vi "VSS_SimulatorCommand.vi"(11 "our_robots":T1[](array[typedef])) -> (2 "Array":u8[](array[numeric]))   [LabVIEW 2017]
uses:
  Core/AI Robot.ctl
  Intel/Functions Enum.ctl
  Intel/AttackerStates.ctl
  Path Planning/RRT/PathDests.ctl
  Path Planning/RRT/PathDest.ctl
panel:
  in  "k":dbl=10.0 format="%#_13g"
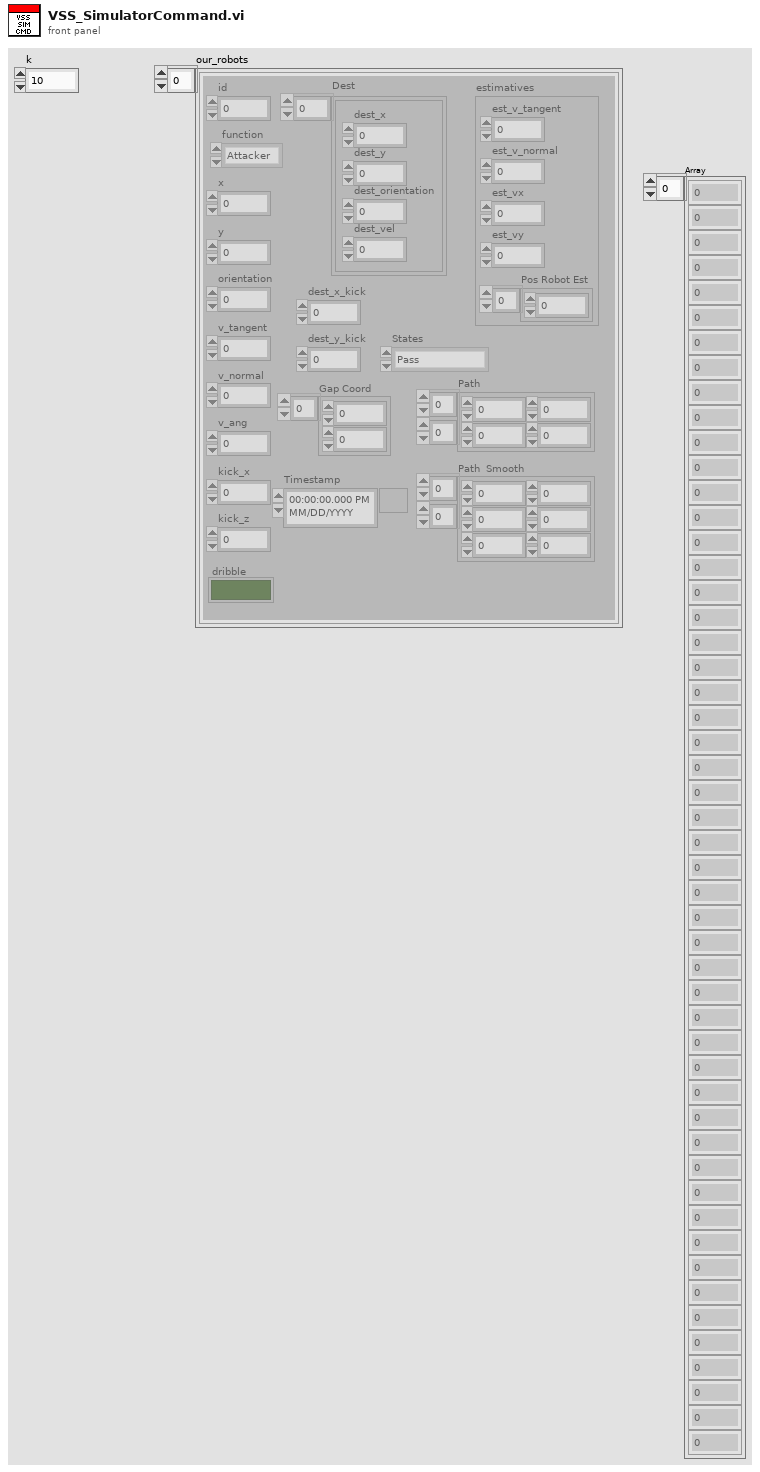
[diagram p1: front panel]
types:
  T1 = typedef "AI Robot.ctl" = cluster{"id":u32, "function":T2, "x":dbl, "y":dbl, "orientation":dbl, "v_tangent":dbl, "v_normal":dbl, "v_ang":dbl, "kick_x":dbl, "kick_z":dbl, "dribble":bool, "Timestamp":timestamp, "estimatives":cluster{"est_v_tangent":dbl, "est_v_normal":dbl, "est_vx":dbl, "est_vy":dbl, "Pos Robot Est":dbl[]}, "dest_x_kick":dbl, "dest_y_kick":dbl, "Gap Coord":dbl[], "States":T3, "Path ":dbl[][], "Path  Smooth":dbl[][], "Dest":T4}
  T2 = typedef "Functions Enum.ctl" = enum16{"Attacker", "Goalie", "Defender", "Striker", "Goto 0", "Dummy", "Kicker", "ZigZag"}
  T3 = typedef "AttackerStates.ctl" = enum16{"Pass", "GoToTangent", "BallGetting", "GoToKick", ""}
  T4 = typedef "PathDests.ctl" = T5[]
  T5 = typedef "PathDest.ctl" = cluster{"dest_x":dbl, "dest_y":dbl, "dest_orientation":dbl, "dest_vel":dbl}
  T6 = typedef "Viewer Robot Command.ctl" = cluster{"Vel Direita 1\n":dbl, "Vel Direita 2":dbl, "Vel Direita 3":dbl, "Vel Esquerda 1\n":dbl, "Vel Esquerda 2":dbl, "Vel Esquerda 3":dbl}
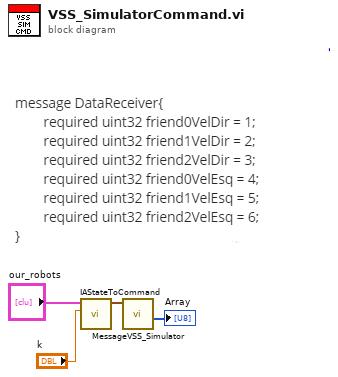
[diagram p0: block diagram]
diagram:
  n1 = call "IAStateToCommand.vi"("k"="k", "our_robots"="our_robots") -> ("Message"=w1:T6)  [unwired: 9 in]
  n2 = call "MessageVSS_Simulator.vi"("Robot"=w1) -> ("Array"=→"Array":u8[])  [unwired: 10 in]
